vi "UARTLoopBackTest.vi"() -> ()   [LabVIEW 2014]
uses:
  <vilib>/Instr/_visa.llb/VISA Configure Serial Port (Instr).vi
panel:
  out "read buffer":string
  out "return count":u32
  out "concatenated string":string
  in  "VISA resource name":refnum<visa-resource-name>
  in  "Loop Timer":u32=500 min=500 max=5000 step=500
  in  "stop":bool
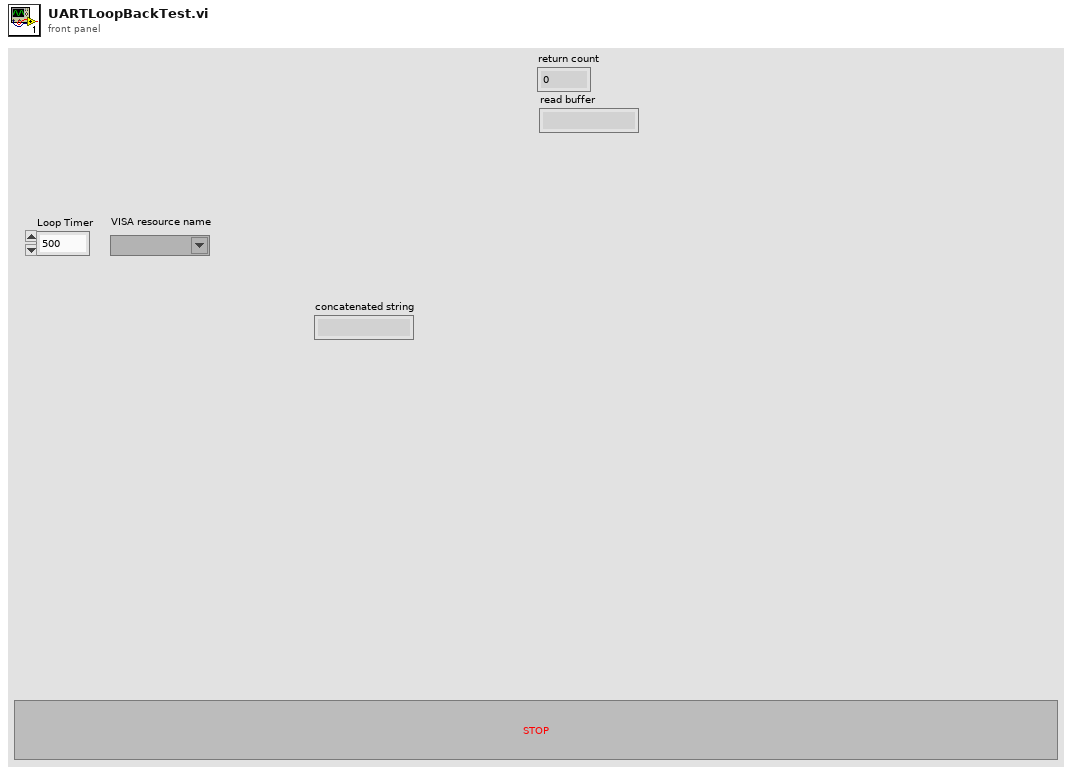
[diagram p1: front panel]
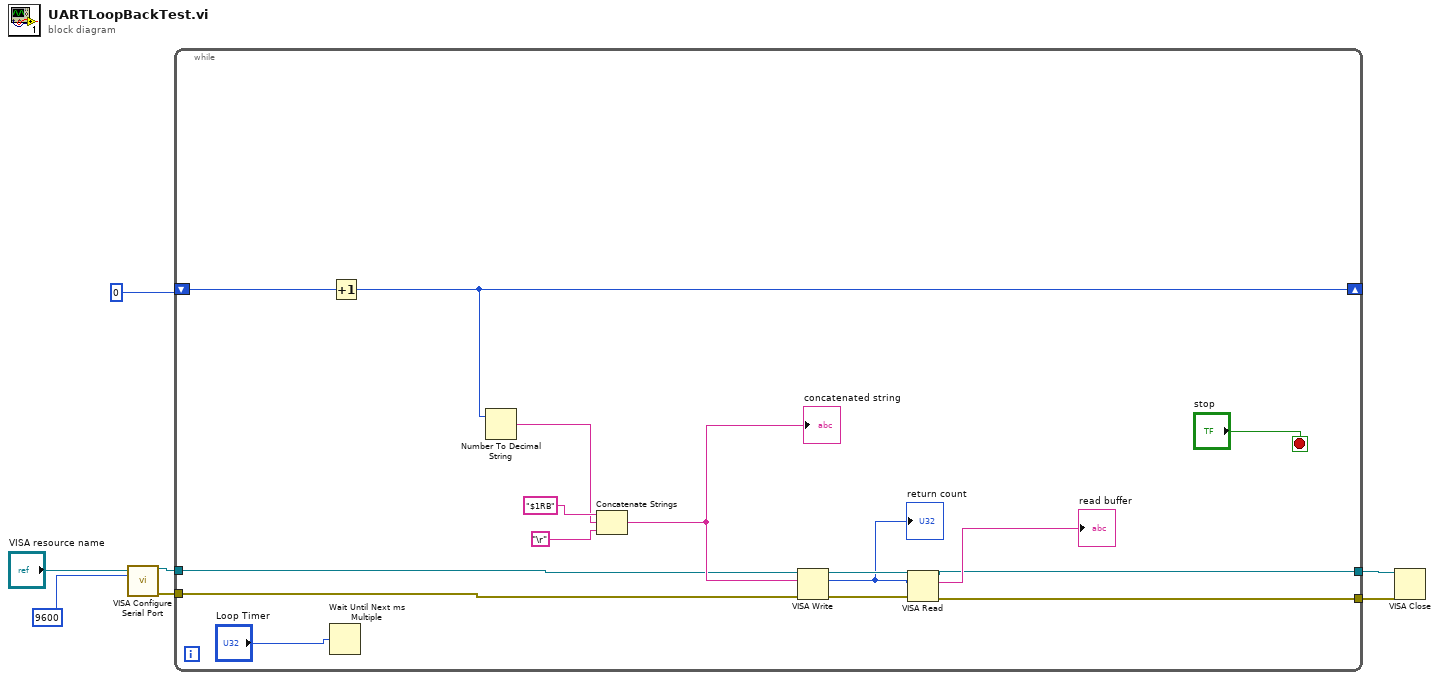
[diagram p0: block diagram]
diagram:
  n1 = call-poly "VISA Configure Serial Port"("VISA resource name"="VISA resource name", "baud rate (9600)"=u32 9600) -> ("VISA resource name out"=w6:refnum<visa-resource-name>, "error out"=w4:errorcluster)  [unwired: 12 in]
  n2 = while {
    tunnel: w6 -> [w15]
    tunnel: w4 -> [w14]
    tunnel: [w9] -> w3
    tunnel: [w8] -> w2
    shift-right: [w18] -> _
    shift-left: 0 -> [w20]
    stop <- "stop" stop-if-true
    n3 = Wait Until Next ms Multiple(millisecond multiple="Loop Timer") -> ()  [unwired: 1 out]
    n4 = Increment(x=w20) -> (x+1=w18:i32)
    n5 = Number To Decimal String(number=w18) -> (decimal integer string=w16:string)  [unwired: 1 in]
    n6 = Concatenate Strings("$1RB", w16, "\r") -> (w22:string)
    "concatenated string" <- w22
    n7 = VISA Write(VISA resource name=w15, write buffer=w22, error in (no error)=w14) -> (VISA resource name out=w12:refnum<visa-resource-name>, return count=w10:u32, error out=w11:errorcluster)
    "return count" <- w10
    n8 = VISA Read(VISA resource name=w12, byte count=w10, error in (no error)=w11) -> (VISA resource name out=w9:refnum<visa-resource-name>, read buffer=→"read buffer":string, error out=w8:errorcluster)  [unwired: 1 out]
  }
  n9 = VISA Close(VISA resource name=w3, error in (no error)=w2) -> ()  [unwired: 1 out]
